vi "slowInterpolationCounter.vi"(7 "reset":bool, 8 "doStep":bool, 11 "upStep":fxp<+,28,0>) -> (2 "fraction":fxp<+,28,0>, 3 "index":u16)   [LabVIEW 2016]
uses:
  <vilib>/rvi/FXPMathLib/FxpAdd/XNode/nifxpmath_Add.xnode
  <vilib>/rvi/FXPMathLib/sim/FxpSim.dll
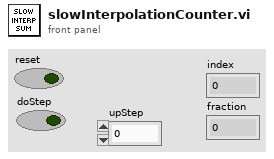
[diagram p1: front panel]
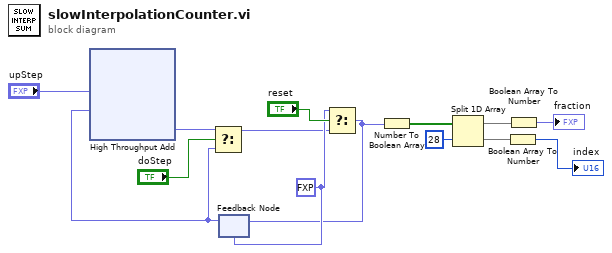
[diagram p0: block diagram]
diagram:
  w11 = fxp<+,42,14> 0.0 ("t")
  n1 = feedback #1(w11) -> (w9:fxp<+,42,14>)
  n2 = xnode ("High Throughput Add")("x"="upStep", "y"=w9) -> ("x+y"=w13:fxp<+,42,14>)
  n3 = Select(t=w13, s="doStep", f=w9) -> (s? t:f=w10:fxp<+,42,14>)
  n4 = Select(t=w11, s="reset", f=w10) -> (s? t:f=w7:fxp<+,42,14>)
  n5 = feedback-in #1(w7) -> ()
  n6 = Number To Boolean Array(number=w7) -> (Boolean array=w6:bool[])
  n7 = Split 1D Array(array=w6, index=28) -> (first subarray=w4:bool[], second subarray=w3:bool[])
  n8 = Boolean Array To Number(Boolean array=w3) -> (number=→"index":u16)
  n9 = Boolean Array To Number(Boolean array=w4) -> (number=→"fraction":fxp<+,28,0>)
